vi "Open file dialog.vi"(8 "error in (no error)":errorcluster, 10 "Default file name":string caption="default name", 11 "File Path Control":path) -> (0 "error out":errorcluster, 2 "File name":string, 3 "selected path":path)   [LabVIEW 2014]
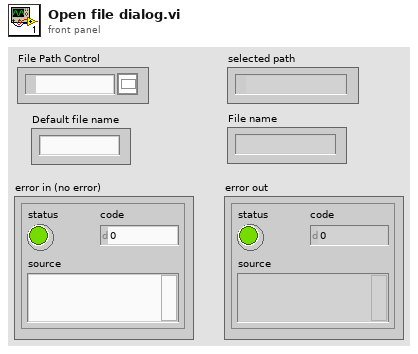
[diagram p1: front panel]
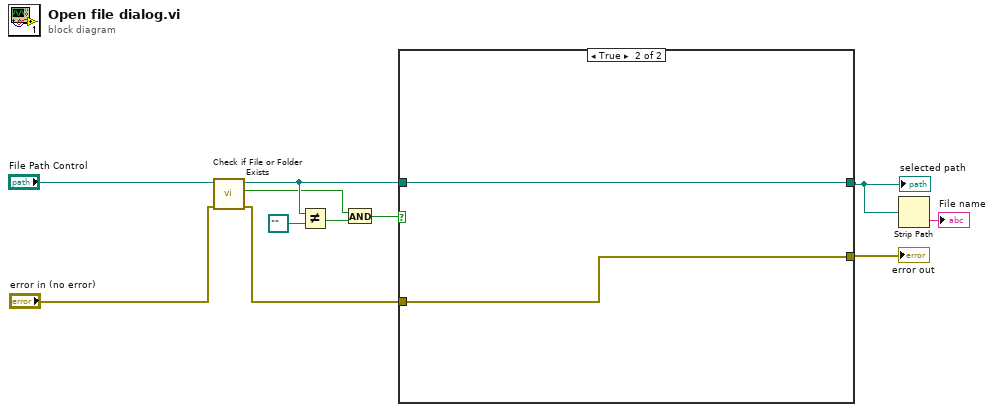
[diagram p0: block diagram]
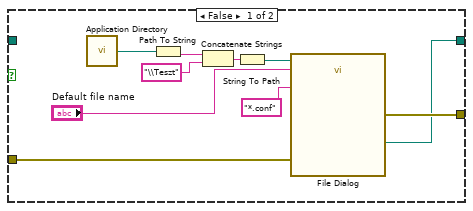
[diagram p2: hidden frame]
diagram:
  n1 = call <vilib>:"Check if File or Folder Exists.vi"("error in (no error)"="error in (no error)", "path"="File Path Control") -> ("error out"=w7:errorcluster, "file or folder exists?"=w2:bool, "dup path"=w5:path)  [unwired: 7 in]
  n2 = Not Equal?(x=w5, y=path "") -> (x != y?=w3:bool)
  n3 = And(x=w2, y=w3) -> (x .and. y?=w1:bool)
  n4 = case shown="True" w1 {
    tunnel: [w21 w23] -> w11
    tunnel: w7 -> [w19 w23]
    tunnel: w5 -> [_ w22]
    tunnel: [w12 w22] -> w6
    frame False {
      n5 = call <vilib>:"Application Directory.vi"() -> ("Application Directory"=w14:path)
      n6 = Path To String(path=w14) -> (string=w18:string)
      n7 = Concatenate Strings(w18, "\\Teszt" ("prompt (Choose or enter file path)")) -> (w17:string)
      n8 = String To Path(string=w17) -> (path=w15:path)
      n9 = call "File Dialog"("start path"=w15, "default name"="Default file name", "error in"=w19, "pattern (all files)"="*.conf") -> ("selected path"=w12:path, "error out"=w21:errorcluster)  [unwired: 8 in, 2 out]
    }
    frame True {
    }
  }
  "selected path" <- w6
  "error out" <- w11
  n10 = Strip Path(path=w6) -> (name=→"File name":string)  [unwired: 1 out]
